vi "ReSize.vi"(11 "Tree in":refnum<class "Tree.lvclass">) -> (3 "Tree out":refnum<class "Tree.lvclass">)   [LabVIEW 2022 SP3, in "Tree.lvclass"]
uses:
  Tree.lvclass
  Tree.lvclass/Tree.ctl
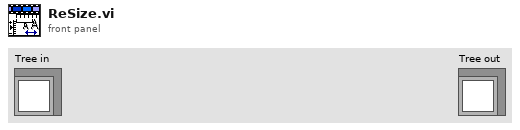
[diagram p1: front panel]
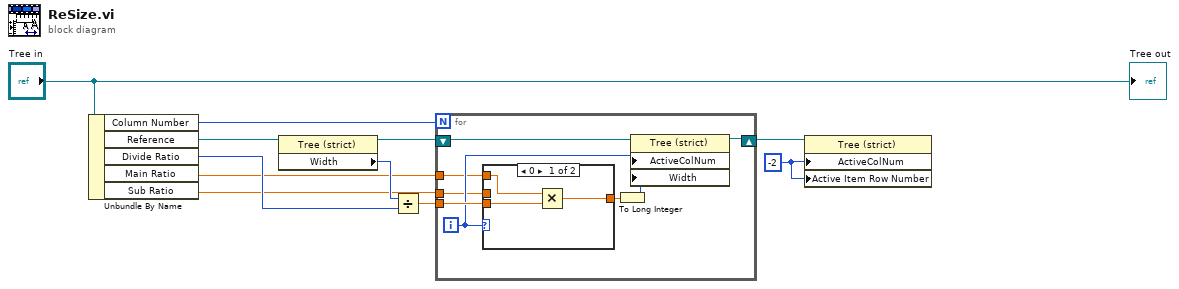
[diagram p0: block diagram]
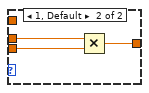
[diagram p2: hidden frame]
diagram:
  w7 = -2 ("Active Cell:Active Column Number")
  n1 = Unbundle By Name("Tree in") -> ("Column Number"=w4:i32, "Reference"=w5:refnum<vi>, "Divide Ratio"=w3:i32, "Main Ratio"=w2:dbl, "Sub Ratio"=w1:dbl)
  n2 = property class="Tree (strict)"(reference=w5) -> (reference out=w10:refnum<vi>, "Width"=w11:u32)  [unwired: 1 in, 1 out]
  n3 = Divide(x=w11, y=w3) -> (x/y=w9:dbl)
  n4 = for {
    N: w4 -> [_]
    shift-right: [w19] -> w8
    shift-left: w10 -> [w18]
    tunnel: w9 -> [w17]
    tunnel: w2 -> [w13]
    tunnel: w1 -> [w12]
    i -> [w16]
    n5 = case shown="0" w16 {
      tunnel: w17 -> [w22 w25]
      tunnel: [w21 w24] -> w15
      tunnel: w13 -> [w20 _]
      tunnel: w12 -> [_ w23]
      frame 0 {
        n6 = Multiply(x=w20, y=w22) -> (x*y=w21:dbl)
      }
      frame 1, Default {
        n7 = Multiply(x=w23, y=w25) -> (x*y=w24:dbl)
      }
    }
    n8 = To Long Integer(number=w15) -> (32bit integer=w14:i32)
    n9 = property class="Tree (strict)"(reference=w18, "ActiveColNum"=w16, "Width"=w14) -> (reference out=w19:refnum<vi>)  [unwired: 1 in, 1 out]
  }
  n10 = property class="Tree (strict)"(reference=w8, "ActiveColNum"=w7, "Active Item Row Number"=w7) -> ()  [unwired: 1 in, 2 out]
  "Tree out" <- "Tree in"
